vi "AppliOffsetsFichAnalog.vi"(3 "entrée d'erreur":errorcluster, 4 "NomProjet":string, 5 "CheminFichier":path) -> (0 "sortie d'erreur":errorcluster, 2 "chemin du fichier en sortie":path)   [LabVIEW 2017]
uses:
  <vilib>/Analysis/baseanly.llb/Mean (DBL).vi
  <vilib>/Waveform/WDTOps.llb/WDT Get Waveform Subset DBL.vi
  <vilib>/Analysis/NI_AALBase.lvlib
panel:
  out "taille(s)":i32
  out "Offset(unités phys)":dbl[](array[numeric])
  out "AutoZero?":bool[](array[boolean])
  out "DebutVoieN":waveform(dbl)(graph)
  out "VoieN":waveform(dbl)(graph)
  out "DonnesOrigine":waveform(dbl)[](graph)
  out "DonnesFinales":waveform(dbl)[](graph)
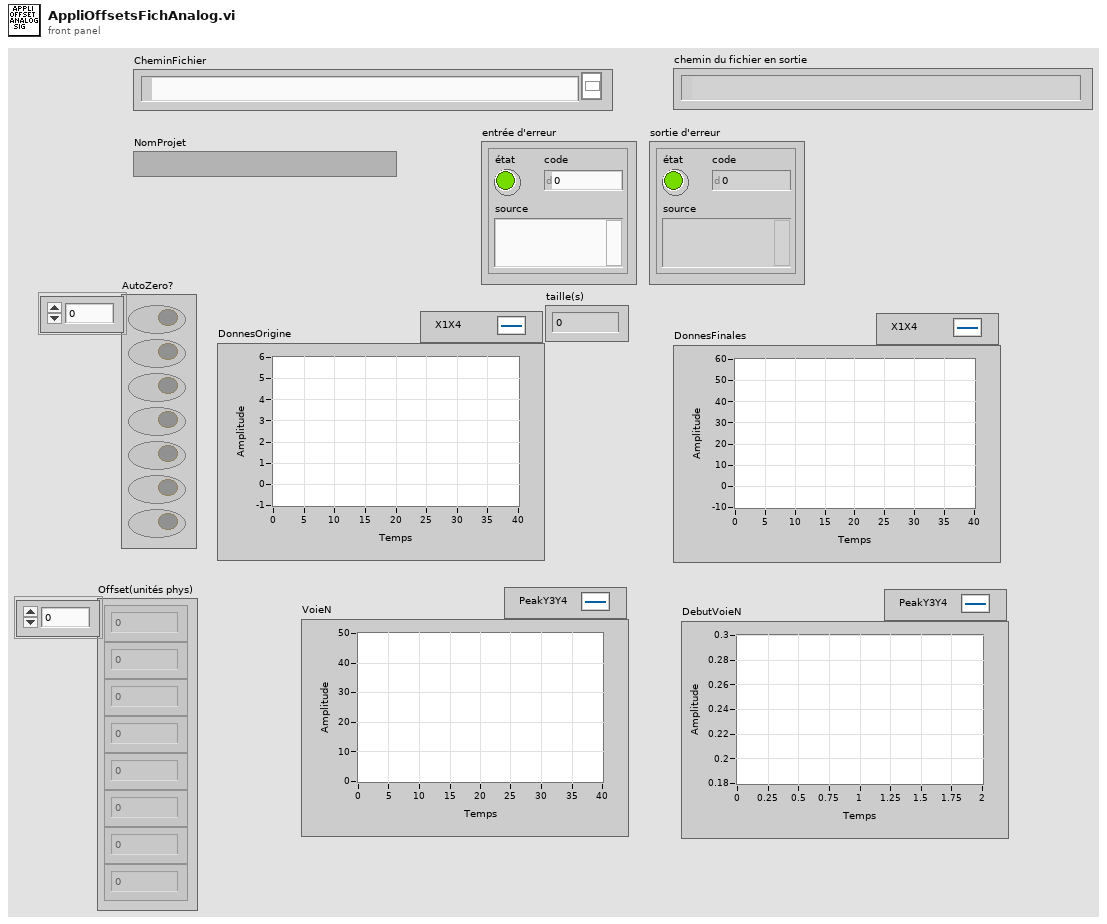
[diagram p1: front panel]
types:
  T1 = enum16{"open", "open or create", "create or replace", "create", "open (read-only)"}
  T2 = typedef "ConfigTotale.ctl" = cluster{"VoltageChannels":T3, "WheastoneBridgeChannels":T4, "Configuration":T5}
  T3 = typedef "VoltageChannels.ctl" = cluster{"ChannelNames":string[], "Sensitivity(Unit/V)":dbl[], "AutoZero":bool[], "ChannelUnits":string[], "Offsets(Units)":dbl[], "Graph Num":u8[]}
  T4 = typedef "WBridgeChannels.ctl" = cluster{"ChannelNames":string[], "Sensitivity(Unit/V)":dbl[], "AutoZero":bool[], "ChannelUnits":string[], "Offsets(Units)":dbl[], "Graph Num":u8[]}
  T5 = typedef "Configuration.ctl" = cluster{"AcqSamplingRate(Hz)":u32, "AcqTime(s)":u32, "Trigger":bool, "NbVoltageChannels":u32, "NbWBridgeChannels":u32, "Qualisys":bool, "Hexapode":bool, "FinalSamplingRate(Hz)":u32, "QualisysDataType":enum16{"6DOF", "3DTracking", "6DOF + 3D"}, "Nortek":bool}
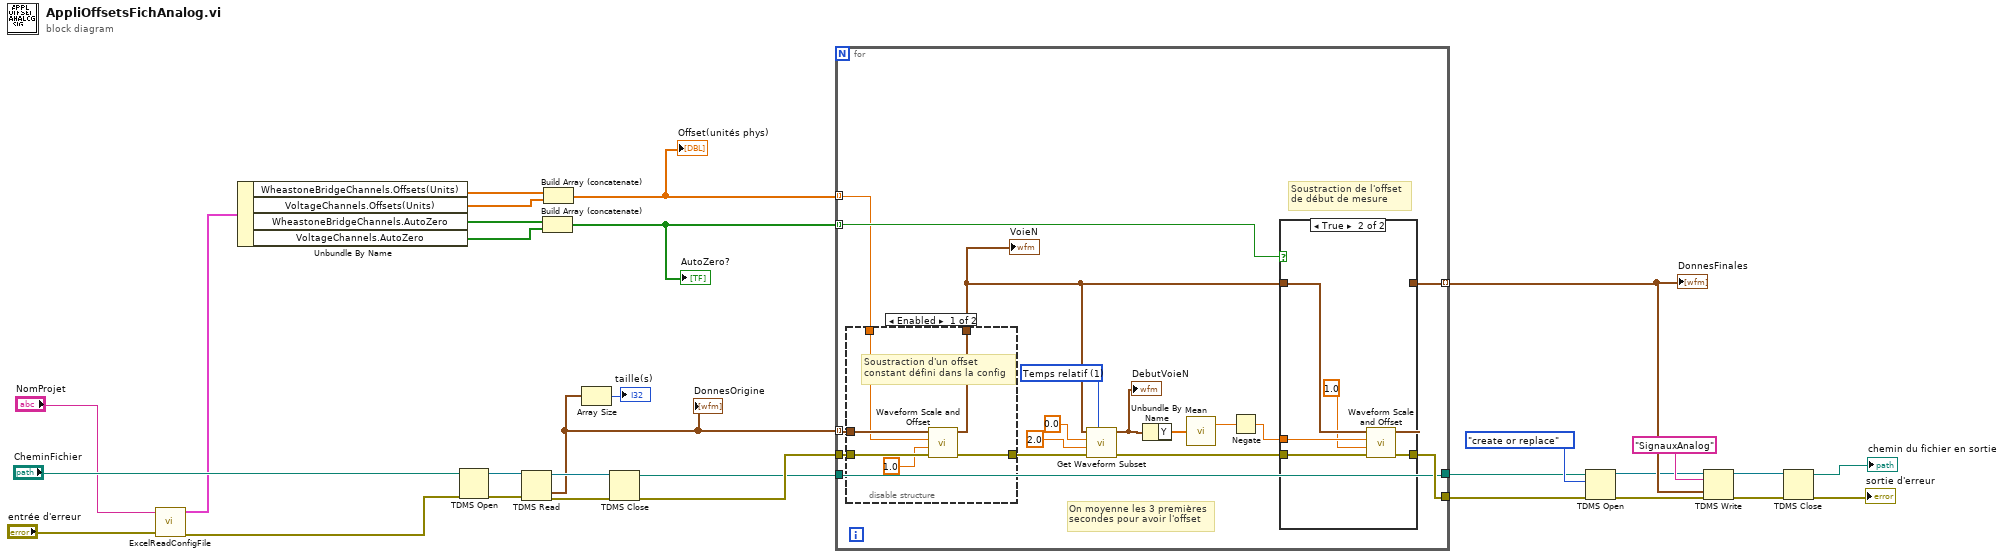
[diagram p0: block diagram]
diagram:
  n1 = call "ExcelReadConfigFile.vi"("NomProjet"="NomProjet", "error in (no error)"="entrée d'erreur") -> ("ConfigurationTotale"=w7:T2, "error out"=w9:errorcluster)  [unwired: 3 in]
  n2 = Unbundle By Name(w7) -> ("WheastoneBridgeChannels.Offsets(Units)"=w6:dbl[], "VoltageChannels.Offsets(Units)"=w5:dbl[], "WheastoneBridgeChannels.AutoZero"=w4:bool[], "VoltageChannels.AutoZero"=w3:bool[])
  n3 = TDMS Open(8:w9, 11:"CheminFichier") -> (0:w18:errorcluster, 3:w17:refnum<k34>)  [unwired: 5 in]
  n4 = TDMS Read(0:w17, 11:w18) -> (4:w24:refnum<k34>, 10:w20:waveform(dbl)[], 15:w23:errorcluster)  [unwired: 6 in, 3 out]
  "DonnesOrigine" <- w20
  n5 = Build Array (concatenate)(w4, w3) -> (w1:bool[])
  "AutoZero?" <- w1
  n6 = Build Array (concatenate)(w6, w5) -> (w2:dbl[])
  "Offset(unités phys)" <- w2
  n7 = Array Size(array=w20) -> (size(s)=→"taille(s)":i32)
  n8 = TDMS Close(8:w23, 11:w24) -> (0:w21:errorcluster, 3:w14:path)
  n9 = for {
    tunnel: w20 -> [w35] mode=indexing
    tunnel: w1 -> [w47] mode=indexing
    tunnel: w21 -> [w37]
    tunnel: [w38] -> w11
    tunnel: [w39] -> w26 mode=indexing
    tunnel: w2 -> [w33] mode=indexing
    tunnel: w14 -> [w32]
    tunnel: [w32] -> w12
    w44 = u16 1 items=["Échantillons", "Temps relatif"] ("start/duration format")
    # "Soustraction de l'offset \nde début de mesure"
    # "On moyenne les 3 premières\nsecondes pour avoir l'offset"
    n10 = disable-structure shown="Enabled" {
      disable-tunnel: w37 -> [w53 w54]
      disable-tunnel: [w52 w54] -> w36
      disable-tunnel: w35 -> [w51 w55]
      disable-tunnel: [w50 w55] -> w34
      disable-tunnel: w33 -> [w49 _]
      frame Enabled {
        # "Soustraction d'un offset\nconstant défini dans la config"
        n11 = call <vilib>:"Waveform Scale and Offset.vi"("error in (no error)"=w53, "scale"=1.0, "offset"=w49, "waveform in"=w51) -> ("error out"=w52:errorcluster, "waveform out"=w50:waveform(dbl))  [unwired: 6 in]
      }
      frame Disabled {
      }
    }
    "VoieN" <- w34
    n12 = call-poly <vilib>:"Get Waveform Subset.vi"("start/duration format"=w44, "error in (no error)"=w36, "duration"=2.0, "start samples/time"=0.0, "waveform in"=w34) -> ("error out"=w43:errorcluster, "waveform out"=w40:waveform(dbl))  [unwired: 1 in, 2 out]
    "DebutVoieN" <- w40
    n13 = Unbundle By Name(w40) -> ("Y"=w31:dbl[])
    n14 = call-poly <vilib>:"Mean.vi"("X"=w31) -> ("mean"=w41:dbl)  [unwired: 1 out]
    n15 = Negate(x=w41) -> (-x=w42:dbl)
    n16 = case shown="True" w47 {
      tunnel: w42 -> [_ w62]
      tunnel: w34 -> [w57 w63]
      tunnel: w43 -> [w56 w60]
      tunnel: [w56 w59] -> w38
      tunnel: [w57 w58] -> w39
      frame False {
      }
      frame True {
        n17 = call <vilib>:"Waveform Scale and Offset.vi"("error in (no error)"=w60, "scale"=1.0, "offset"=w62, "waveform in"=w63) -> ("error out"=w59:errorcluster, "waveform out"=w58:waveform(dbl))  [unwired: 6 in]
      }
    }
  }
  "DonnesFinales" <- w26
  n18 = TDMS Open(8:w11, 10:T1."create or replace" ("opération (0 : open)"), 11:w12) -> (0:w15:errorcluster, 3:w16:refnum<k34>)  [unwired: 4 in]
  n19 = TDMS Write(0:w16, 5:"SignauxAnalog" ("nom du groupe en entrée (Sans titre)"), 9:w26, 11:w15) -> (4:w30:refnum<k34>, 15:w29:errorcluster)  [unwired: 2 in, 2 out]
  n20 = TDMS Close(8:w29, 11:w30) -> (0:→"sortie d'erreur":errorcluster, 3:→"chemin du fichier en sortie":path)
